vi "Coordinate_Trans_.vi"(3 "Simulate/Run":T1, 4 "Input Position":dbl[](array[numeric])=[0.0, 0.0, 0.0] format="%.2f", 5 "Traverse Name":string) -> (0 "Z":dbl, 1 "Y":dbl, 2 "X":dbl)   [LabVIEW 2015]
uses:
  Controls/User_Specific_mode.ctl
  Controls/Tunnel_Coordinates.ctl
  ADAM Client/Sub VIs/ADAM Controls/Quick_local_ADAM_Table.ctl
  Globals/Trav_pos_global.vi
  Globals/Extra_Commands_Global.vi
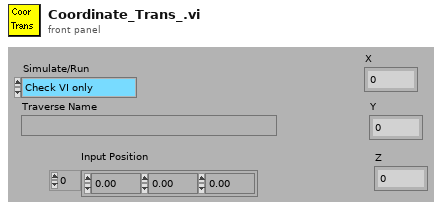
[diagram p1: front panel]
types:
  T1 = typedef "User_Specific_mode.ctl" = enum16{"Check VI only", "Run VI"}
  T2 = typedef "Traverse_cluster.ctl" = cluster{"Start X":sgl, "Start Y":sgl, "Start Z":sgl, "End X":sgl, "End Y":sgl, "End Z":sgl, "No. of pts.":i32, "Spacing":T3, "Filename":path, "Tunnel Speed":dbl, "Averaging time (min)":dbl, "Extra Commands":string, "Carrier_1 Q (l/min)":dbl, "Carrier_2 Q (l/min)":dbl, "Trace Gas Concentration (%)":dbl, "Specific Arguments":string, "Comments":string, "Row No":i32, "Row Type Selector":T4, "Completion time":string, "Row Duration (mins)":dbl, "No. of Valid pts.":i32, "Meas Setup File":string}
  T3 = typedef "Spacing.ctl" = enum16{"Linear", "Log", "Gauss", "Specified", "N/A"}
  T4 = typedef "Multi_run_mode.ctl" = enum16{"Move Traverse Only", "Set Tunnel Speed Only", "Set Source Only", "Set Measurement Conditions", "Single Measurement", "Vertical Profile", "Lateral Profile", "Longitudinal Profile", "Explore Volume", "Multi-Axis Profile", "Auto Calibrate", "Meas Fast FID Bkgnd", "Check Beam Power", "Scanning Valve Measurement", "Run VI Named:", "Set ADAM Ch", "Wait (minutes)", "Send Message", "Synchronize With:", "Fall Back to this Row", "Turn Off Row Repeating", "Blank Row", "Traverse 3D Volume"}
  T5 = typedef "Tunnel_Coordinates.ctl" = enum16{"Work in Tunnel Coordinates", "Work in Model Coordinates"}
  T6 = enum16{"To Traverse Coordinates", "To User Coordinates"}
  T7 = typedef "Quick_local_ADAM_Table.ctl" = enum16{"Read Global", "Load Global From ADAM Table", "Write Global"}
  T8 = cluster{"Input Position[0]":dbl, "Input Position[1]":dbl, "Input Position[2]":dbl}
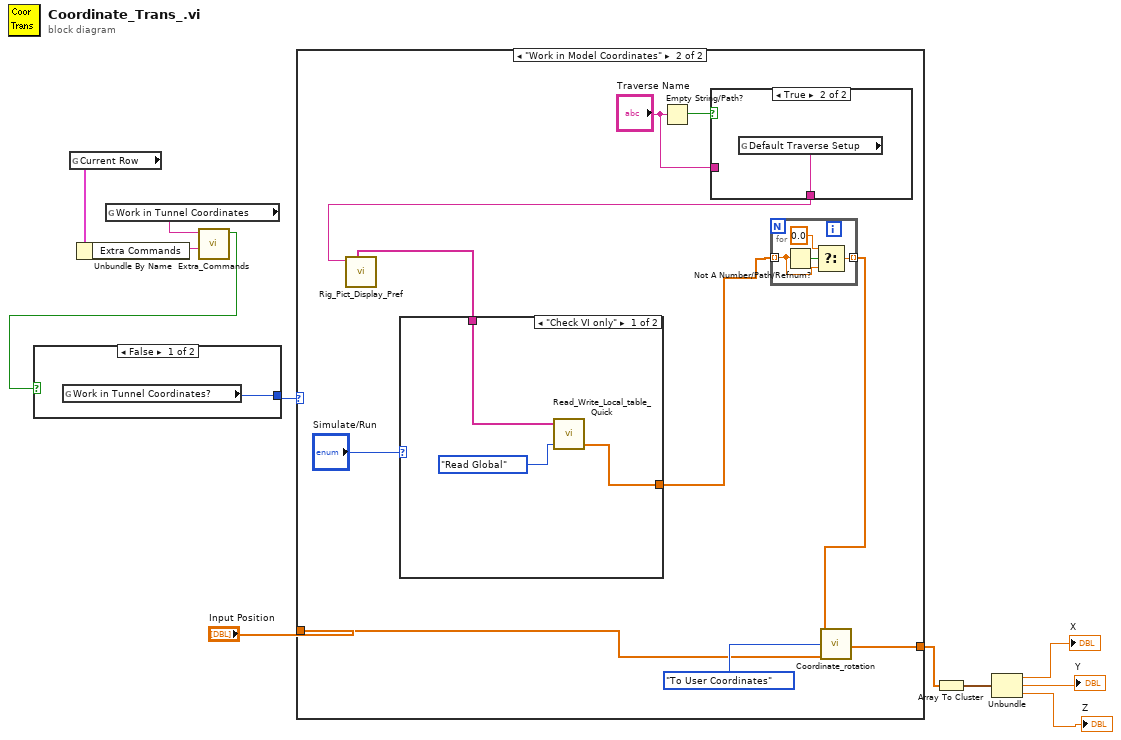
[diagram p0: block diagram]
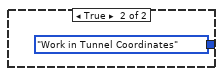
[diagram p2: hidden frame]
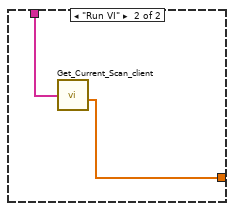
[diagram p4: hidden frame]
diagram:
  n1 = global read "Trav_pos_global.vi" "Current Row"() -> (w3:T2)
  n2 = Unbundle By Name(w3) -> ("Extra Commands"=w4:string)
  n3 = global read "Extra_Commands_Global.vi" "Work in Tunnel Coordinates"() -> (w5:string)
  n4 = call "Extra_Commands.vi"("String to Search"=w4, "Command"=w5) -> ("Command Found"=w2:bool)  [unwired: 1 in, 4 out]
  n5 = case shown="False" w2 {
    tunnel: [w12 Tunnel_Coordinates."Work in Tunnel Coordinates" ("Work in Tunnel Coordinates?")] -> w1
    frame False {
      n6 = global read "Trav_pos_global.vi" "Work in Tunnel Coordinates?"() -> (w12:T5)
    }
    frame True {
    }
  }
  n7 = case shown="\"Work in Model Coordinates\"" w1 {
    tunnel: [w14 w22] -> w9
    tunnel: "Input Position" -> [w14 w23]
    frame "Work in Tunnel Coordinates" {
    }
    frame "Work in Model Coordinates" {
      n8 = Empty String/Path?(string/path="Traverse Name") -> (empty?=w20:bool)
      n9 = case shown="True" w20 {
        tunnel: [w30 w31] -> w19
        tunnel: "Traverse Name" -> [w30 _]
        frame False {
        }
        frame True {
          n10 = global read "Trav_pos_global.vi" "Default Traverse Setup"() -> (w31:string)
        }
      }
      n11 = call "Rig_Pict_Display_Pref.vi"("Traverse Name"=w19) -> ("Roll Pitch Yaw ADAM Channels"=w17:string[])  [unwired: 3 in, 4 out]
      n12 = case shown="\"Check VI only\"" "Simulate/Run" {
        tunnel: [w25 w28] -> w16
        tunnel: w17 -> [w26 w29]
        frame "Check VI only" {
          n13 = call "Read_Write_Local_table_Quick.vi"("Mode"=Quick_local_ADAM_Table."Read Global", "Ch names In"=w26) -> ("Numeric Values Out"=w25:dbl[])  [unwired: 1 in, 2 out]
        }
        frame "Run VI" {
          n14 = call "Get_Current_Scan_client.vi"("ADAM Ch Names"=w29) -> ("Numerical Values"=w28:dbl[])  [unwired: 3 out]
        }
      }
      n15 = for {
        tunnel: w16 -> [w34] mode=indexing
        tunnel: [w32] -> w21 mode=indexing
        n16 = Not A Number/Path/Refnum?(number/path/refnum=w34) -> (NaN/Path/Refnum?=w35:bool)
        n17 = Select(t=0.0, s=w35, f=w34) -> (s? t:f=w32:dbl)
      }
      n18 = call "Coordinate_rotation.vi"("Roll-Pitch-Yaw"=w21, "Input Position"=w23, "Mode"=T6."To User Coordinates") -> ("Output Position"=w22:sgl[])  [unwired: 2 in, 1 out]
    }
  }
  n19 = Array To Cluster(array=w9) -> (cluster=w10:T8)
  n20 = Unbundle(w10) -> ("Input Position[0]"=→"X":dbl, "Input Position[1]"=→"Y":dbl, "Input Position[2]"=→"Z":dbl)
